vi "layline.vi"(11 "Boat Direction":dbl(knob) scale=0.0..360.0) -> (3 "Layline Direction":dbl(knob) scale=0.0..360.0)   [LabVIEW 2013]
doc: "The layline is at a right angle to the boat in an upwind direction\n\nKaitlin"
panel:
  in  "Absolute Wind Direction":dbl(knob) scale=0.0..360.0
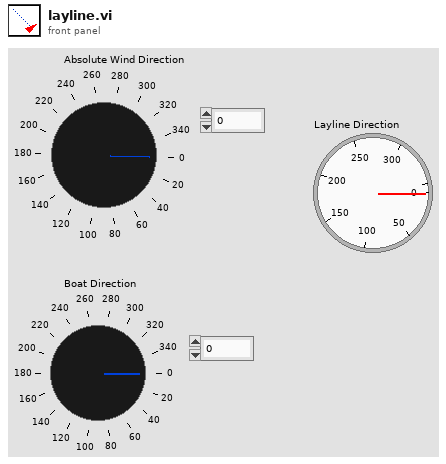
[diagram p1: front panel]
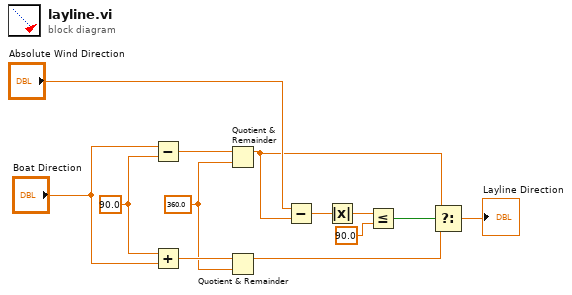
[diagram p0: block diagram]
diagram:
  w9 = 360.0
  w12 = 90.0
  n1 = Subtract(x="Boat Direction", y=w12) -> (x-y=w11:dbl)
  n2 = Add(x=w12, y="Boat Direction") -> (x+y=w10:dbl)
  n3 = Quotient & Remainder(x=w11, y=w9) -> (x-y*floor(x/y)=w3:dbl)  [unwired: 1 out]
  n4 = Quotient & Remainder(x=w10, y=w9) -> (x-y*floor(x/y)=w2:dbl)  [unwired: 1 out]
  n5 = Subtract(x="Absolute Wind Direction", y=w3) -> (x-y=w7:dbl)
  n6 = Absolute Value(x=w7) -> (abs(x)=w6:dbl)
  n7 = Less Or Equal?(x=w6, y=90.0) -> (x <= y?=w4:bool)
  n8 = Select(t=w3, s=w4, f=w2) -> (s? t:f=→"Layline Direction":dbl)
